vi "Read Config File Path.vi"(8 "error in (no error)":errorcluster, 11 "Process In":refnum<class "Base.lvclass">) -> (0 "error out":errorcluster, 2 "Config File Path":path, 3 "Process Out":refnum<class "Base.lvclass">)   [LabVIEW 2020, in "Base.lvclass"]
doc: "Read the configuration file path used by the class and specified during initialization. If nothing was specified, the default configuration file path is returned."
uses:
  Base.lvclass
  Base.lvclass/Base.ctl
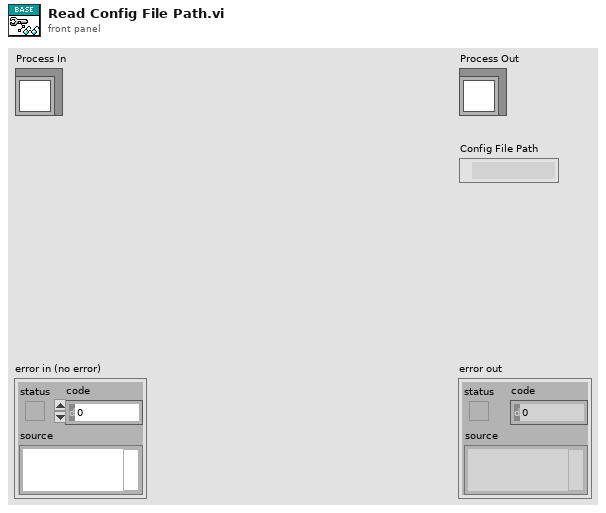
[diagram p1: front panel]
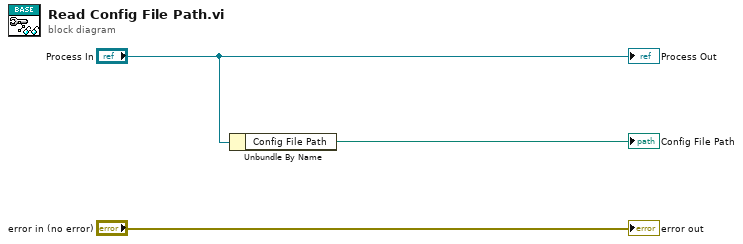
[diagram p0: block diagram]
diagram:
  n1 = Unbundle By Name("Process In") -> ("Config File Path"=→"Config File Path":path)
  "error out" <- "error in (no error)"
  "Process Out" <- "Process In"
